vi "DB - [AMS].[Config].[MessageTemplate].vi"(0 "connection reference":T5, 1 "DB Connection":T6={"Open"=TRUE, "Close"=TRUE}, 2 "Simulate Parameters":T1={"Simulate Send SMS"=TRUE, "Simulate Stringx [Unicode]"=FALSE, "Simulate Send Email"=FALSE, "Simulate Email Fail"=FALSE, "Simulate SMS Fail"=FALSE}, 3 "AMS General Settings":T2, 5 "AMS.Execute.Message":string[](array[string]), 9 "AMS Execute Message ColNames":T4[](array[typedef])=[enum."[MessageNo]", enum."[LanguageId]", enum."[SoftwareSolutionId]", enum."[SoftwareSolutionName]", enum."[PlantId]", enum."[SystemId]", enum."[StationId]", enum."[MessageLogNo]", enum."[ReceivedOn]", enum."[MessageCode]", enum."[ShortDescription]", enum."[Message]", enum."[SmsMessage]", enum."[TransactionNo]", enum."[TransactionRunNo]", enum."[MessageInitiator]", enum."[Remarks]", enum."[MsgCreatedOn]", enum."[IsToSendSms]", enum."[IsToSendEmail]", enum."[SmsContent]", enum."[EmailContent]", enum."[MobileNos]", enum."[EmailAddresses]", enum."[LastAttemptedCommMed]", enum."[LastAttemptedNo]", enum."[IsSmsSent]", enum."[IsEmailSent]", enum."[OverallSentStatus]", enum."[IsArchived]"], 11 "error in (no error)":errorcluster, 12 "[CommMediumId]":string="2", 14 "AMS Configure Parameters":T3) -> (4 "connection reference":T5, 6 "AMS.Config.MessageTemplate":string[](array[string]), 8 "All SMS/Email Delivered OK":bool, 15 "SUMMARY":errorcluster)   [LabVIEW 2013]
uses:
  <vilib>/addons/database/Connection.llb/Conn ObjectReference.ctl
  Controls/DB - OpenClose.ctl
  Controls/DB - [AMS].[Execute].[Message] ColNames.ctl
  Controls/Configure Parameters - AMS.ctl
  Controls/General Settings - AMS.ctl
  Controls/Simulate Parameters - AMS.ctl
  Controls/DB - [AMS].[Execute].[Message] Enum.ctl
  Controls/Global AMS.vi
  Controls/Global SRTRS.vi
  <vilib>/addons/database/Connection.llb/DB Tools Open Connec (String).vi
  tool_Unicode_Convert Unicode to ASCII (Scalar).vi
  <vilib>/addons/database/NI_Database_API.lvlib
panel:
  out "Email Subject (ASCII)":string
  out "AMS.Execute.MessageProcessLog 2":errorcluster
  out "AMS.Execute.Message":errorcluster
  out "AMS.Execute.SmsRefNoLogRelation":errorcluster
  out "[MessageNo]":string
  out "Final Message Delivered OK":bool[](array[boolean])
  in  "AMS.Execute.SmsRefNoLogRelation":string="AMS.Execute.SmsRefNoLogRelation"
  out "AMS.Execute.MessageProcessLog":errorcluster
  in  "AMS.Execute.MessageProcessLog":string="AMS.Execute.MessageProcessLog"
  out "SMS":errorcluster
  out "Email":errorcluster
  out "Message Delivered OK":bool
  in  "Simulate Stringx [Unicode]":string="°e RaW"
  out "SMSString":string
  out "[MessageTemplate.Subject] Unicode":string
  out "EmailAddresses":string[](array[string])
  out "AMS.Config.CommDevice":errorcluster
  out "AMS.Config.CommDeviceCountry":errorcluster
  in  "AMS.Config.CommDevice":string="AMS.Config.CommDevice"
  out "MobileNo/Email, CommDeviceId":string[][](array[string])
  out "MobileNos":string[](array[string])
  out "AMS.Config.CommDeviceCountry":string[][](array[string])
  in  "AMS.Config.CommDeviceCountry":string="AMS.Config.CommDeviceCountry"
  out "SQL":string[](array[string])
  out "AMS.Config.MessageTemplate":errorcluster
  out "AMS.Config.Language":errorcluster
  out "Stringx [Unicode]":string
  out "[IsUnicode]":bool
  in  "AMS.Config.Language":string="AMS.Config.Language"
  out "[SoftwareSolutionId]":string
  out "Close":errorcluster
  out "[LanguageId]":string
  in  "AMS.Config.MessageTemplate":string="AMS.Config.MessageTemplate"
  out "Connection Information":T7={"Connection "="SQL Server 32bit HPEnvy", "Username"="admin", "Password"="admin123"}
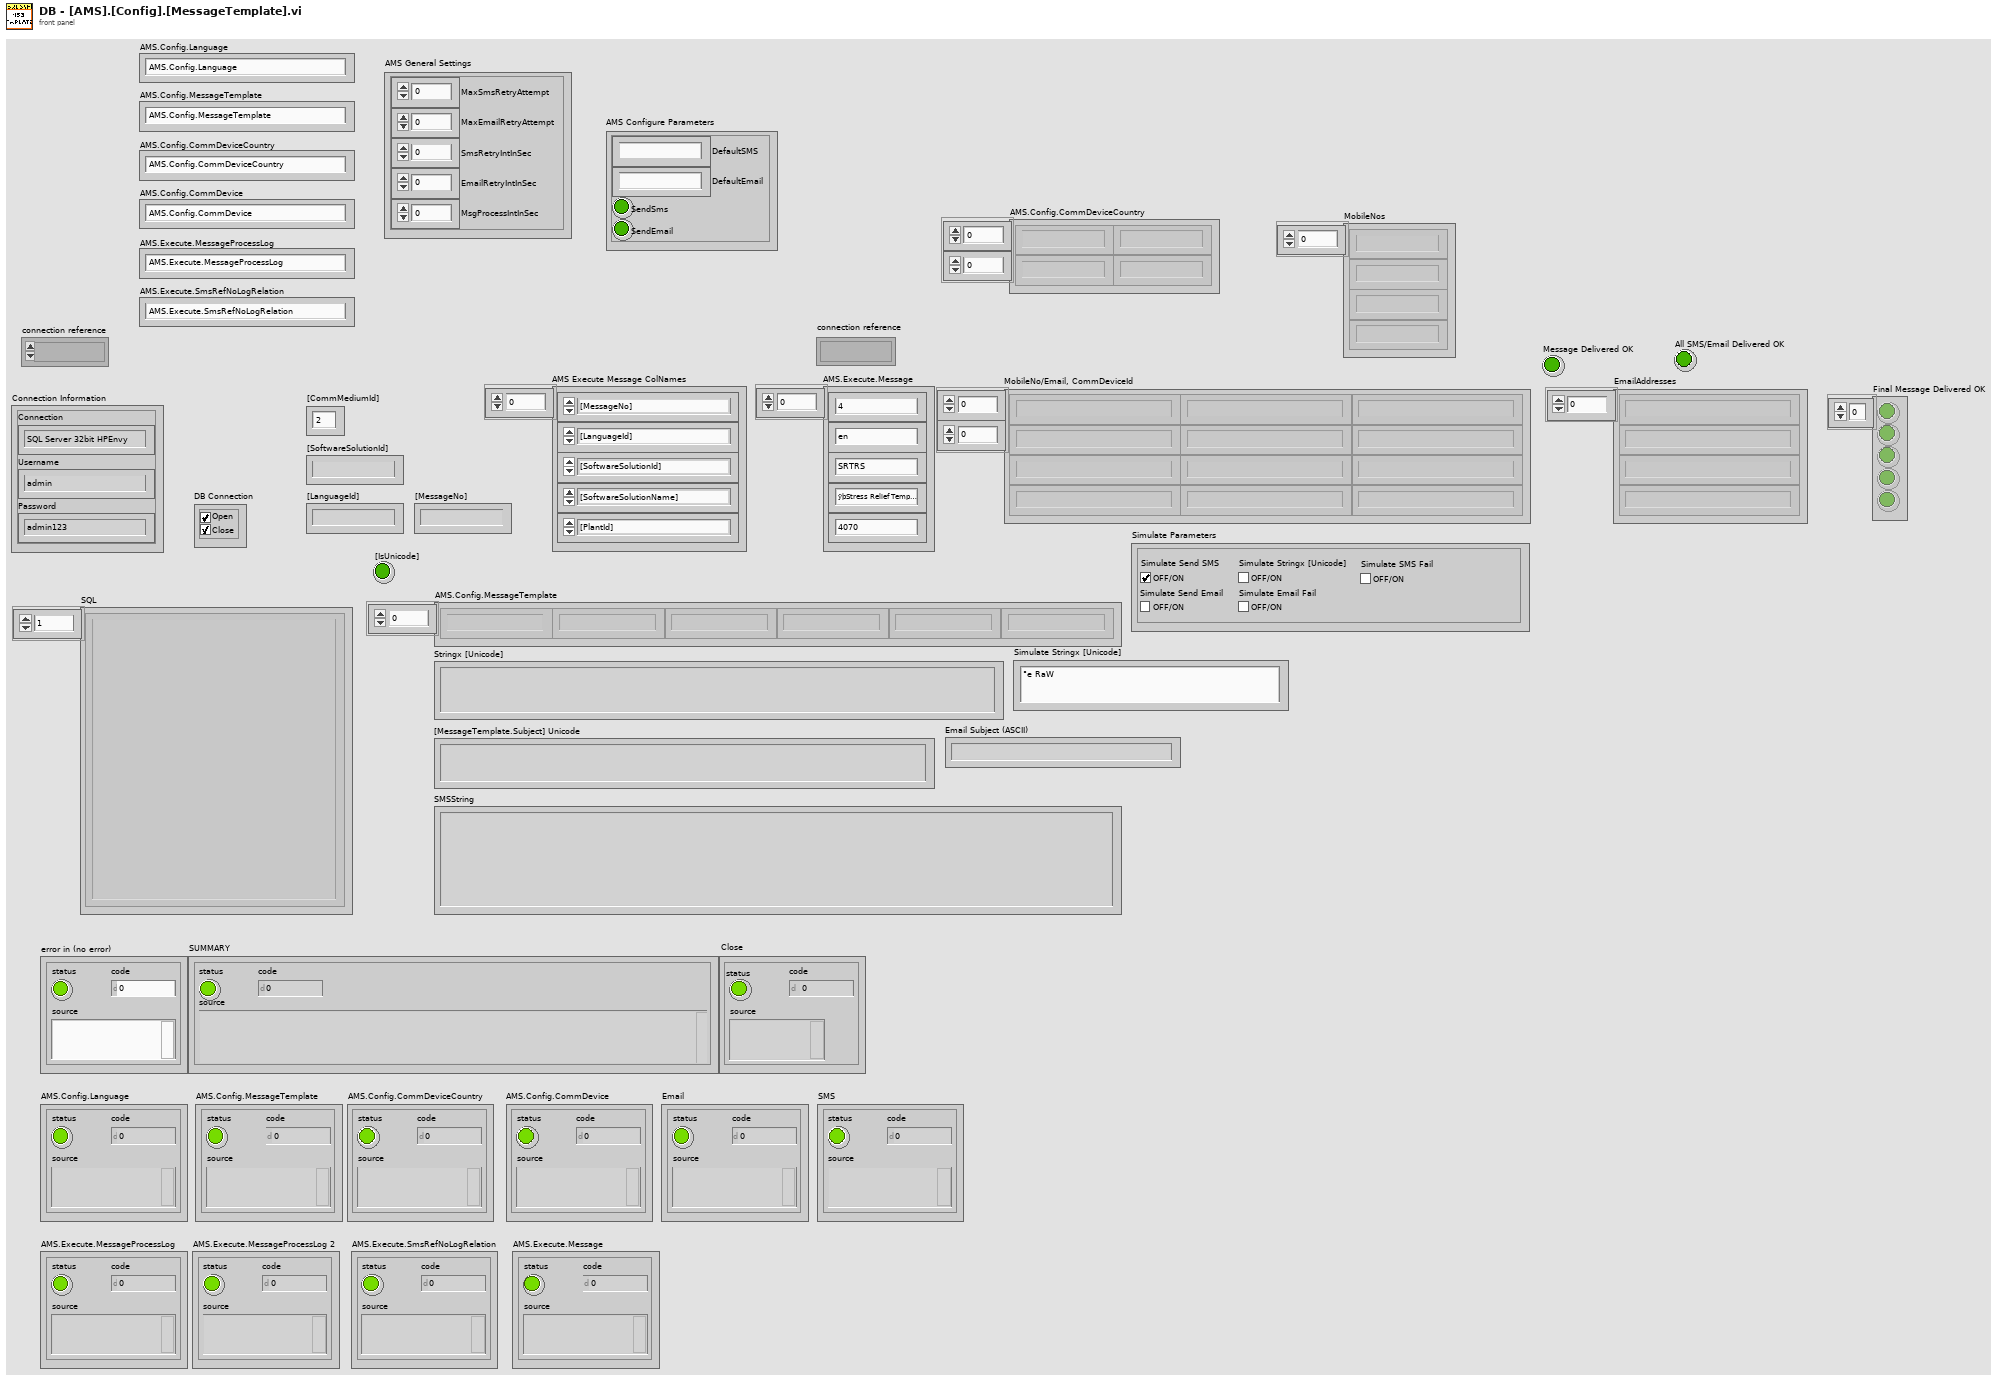
[diagram p1: front panel]
types:
  T1 = typedef "Simulate Parameters - AMS.ctl" = cluster{"Simulate Send SMS":bool, "Simulate Stringx [Unicode]":bool, "Simulate Send Email":bool, "Simulate Email Fail":bool, "Simulate SMS Fail":bool}
  T2 = typedef "General Settings - AMS.ctl" = cluster{"MaxSmsRetryAttempt":i32, "MaxEmailRetryAttempt":i32, "SmsRetryIntInSec":i32, "EmailRetryIntInSec":i32, "MsgProcessIntInSec":i32}
  T3 = typedef "Configure Parameters - AMS.ctl" = cluster{"DefaultSMS":string, "DefaultEmail":string, "SendSms":bool, "SendEmail":bool}
  T4 = typedef "DB - [AMS].[Execute].[Message] ColNames.ctl" = enum16{"[MessageNo]", "[LanguageId]", "[SoftwareSolutionId]", "[SoftwareSolutionName]", "[PlantId]", "[SystemId]", "[StationId]", "[MessageLogNo]", "[ReceivedOn]", "[MessageCode]", "[ShortDescription]", "[Message]", "[SmsMessage]", "[SuppMessage1]", "[SuppMessage2]", "[SuppMessage3]", "[TransactionNo]", "[TransactionRunNo]", "[MessageInitiator]", "[Remarks]", "[MsgCreatedOn]", "[IsToSendSms]", "[IsToSendEmail]", "[IsToSendCommMedium1]", "[IsToSendCommMedium2]", "[SmsContent]", "[EmailContent]", "[CommMed1Content]", "[CommMed2Content]", "[MobileNos]", "[EmailAddresses]", "[CommMedium1Ids]", "[CommMedium2Ids]", "[LastAttemptedCommMed]", "[LastAttemptedNo]", "[LastAttemptedOn]", "[IsSmsSent]", "[IsEmailSent]", "[IsCommMedium1Sent]", "[IsCommMedium2Sent]", "[OverallSentStatus]", "[StatusUpdatedOn]", "[IsArchived]"}
  T5 = typedef "NI_Database_API.lvlib/Conn ObjectReference.ctl" = refnum<k1>
  T6 = typedef "DB - OpenClose.ctl" = cluster{"Open":bool, "Close":bool}
  T7 = cluster{"Connection ":string, "Username":string, "Password":string}
  T8 = typedef "Enum - InteractiveMode-SubVIMode.ctl" = enum16{"Interactive", "subVI Mode"}
  T9 = typedef "Connection Information Cluster.ctl" = cluster{"Connection ":string, "Username":string, "Password":string}
  T10 = typedef "DB - DB.Schema.Table.ctl" = cluster{"DB":string, "Schema":string, "Table":string}
  T11 = typedef "DB - [AMS].[Execute].[Message] Enum.ctl" = enum16{"SELECT", "SELECT (Multi-Conditions)", "UPDATE", "RE-INSERT"}
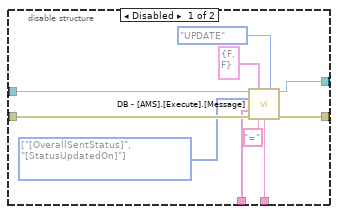
[diagram p2: hidden frame]
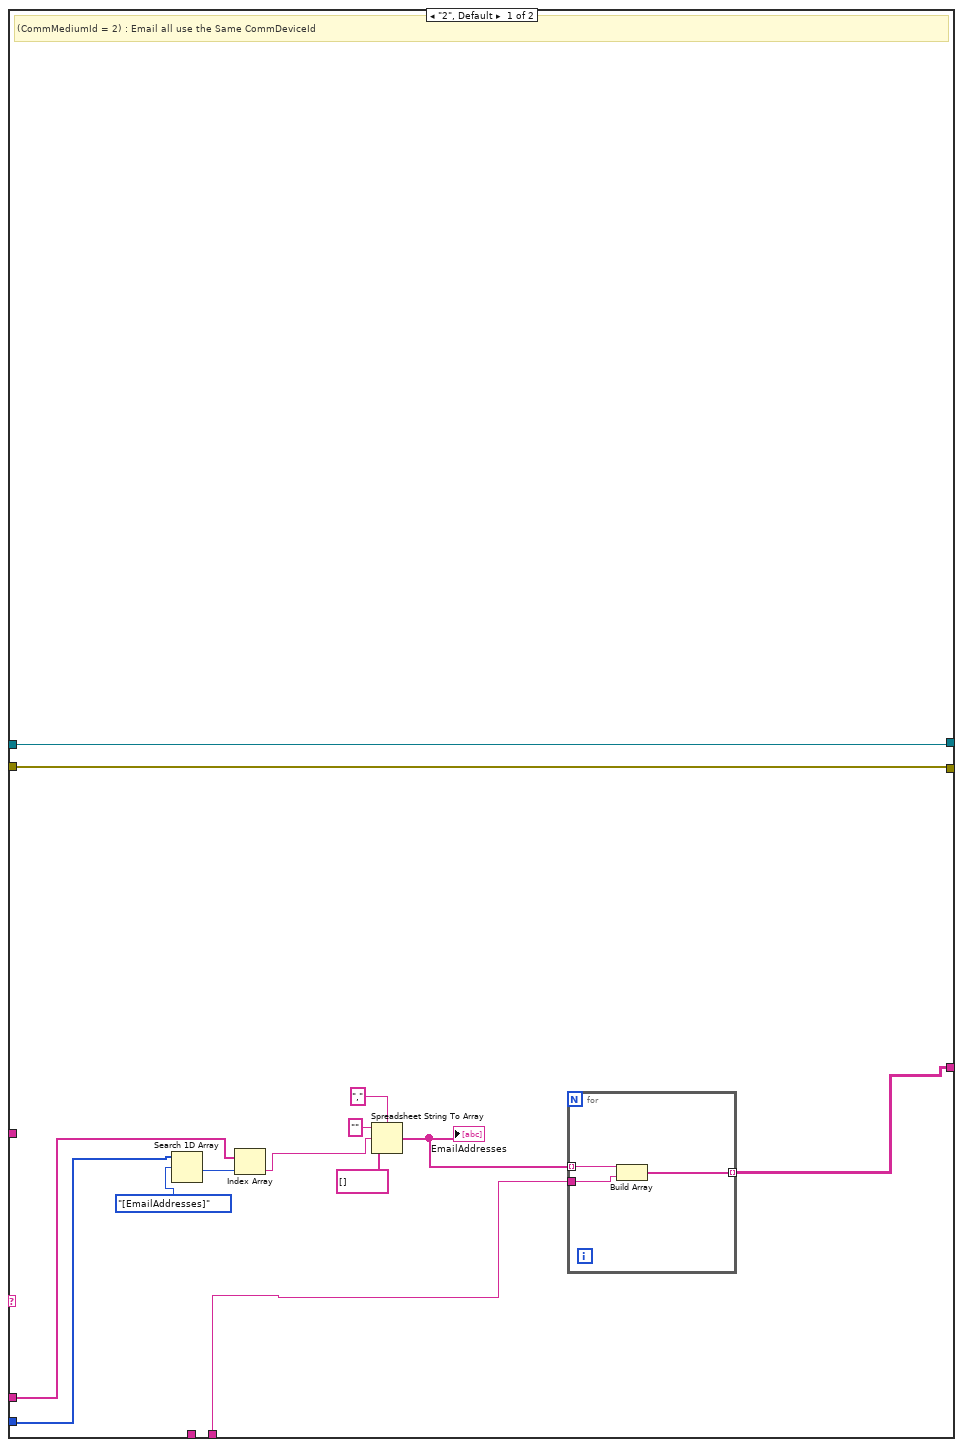
[diagram p3: hidden frame]
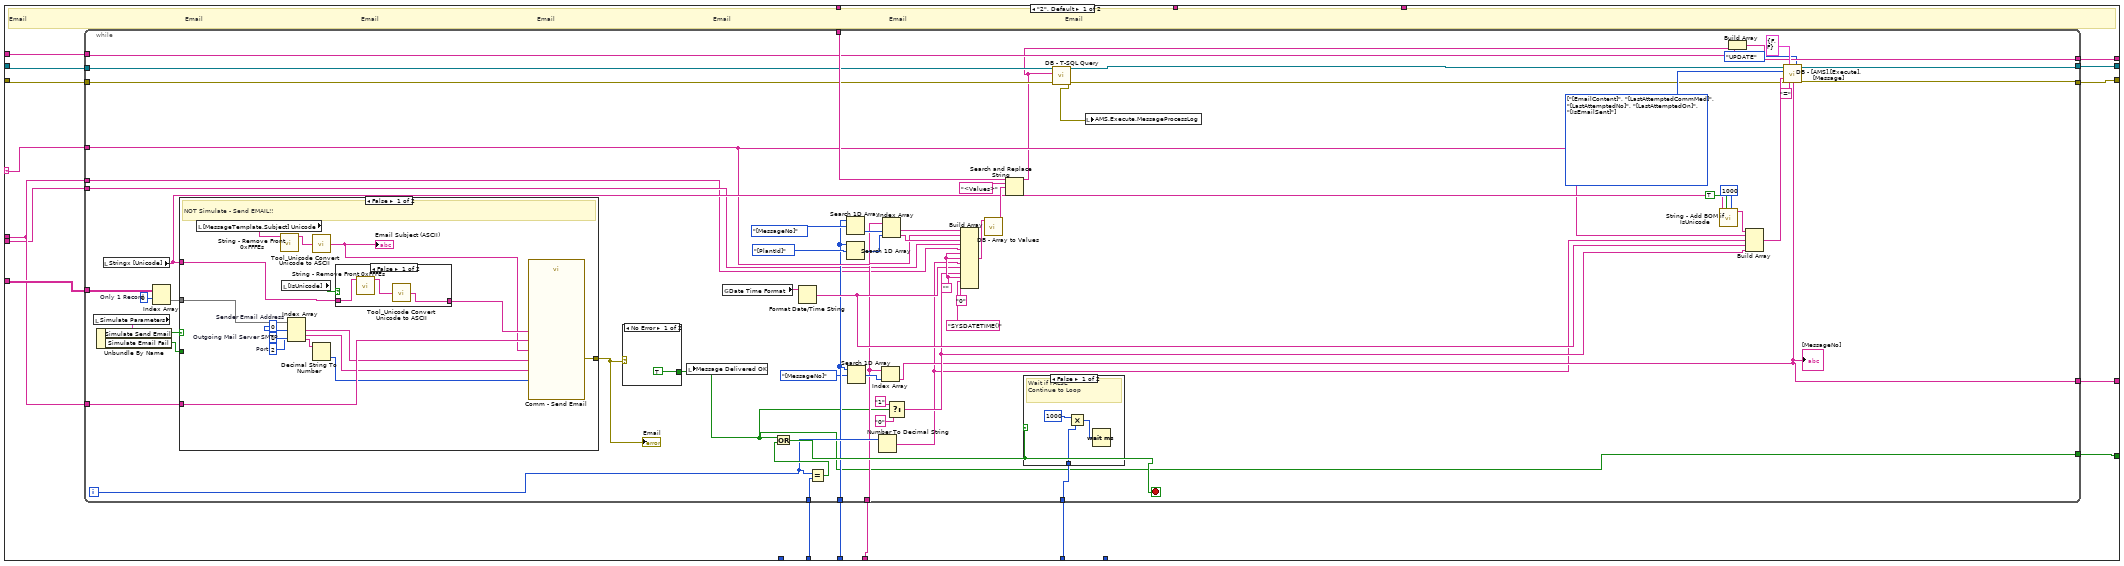
[diagram p4: hidden frame]
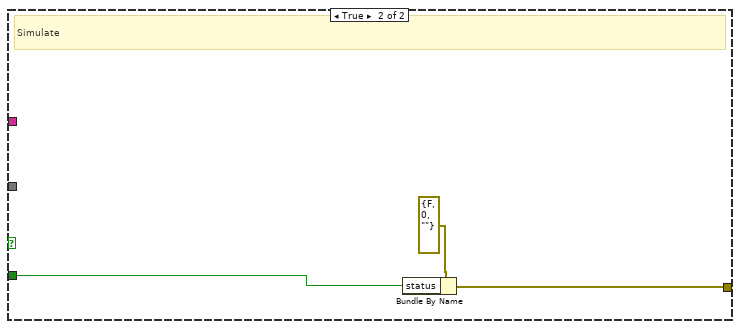
[diagram p6: hidden frame]
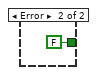
[diagram p8: hidden frame]
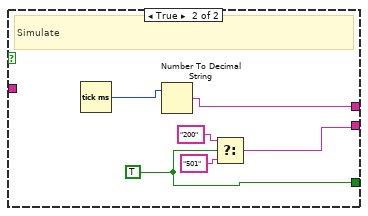
[diagram p10: hidden frame]
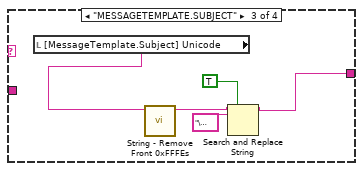
[diagram p13: hidden frame]
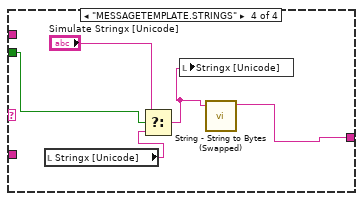
[diagram p14: hidden frame]
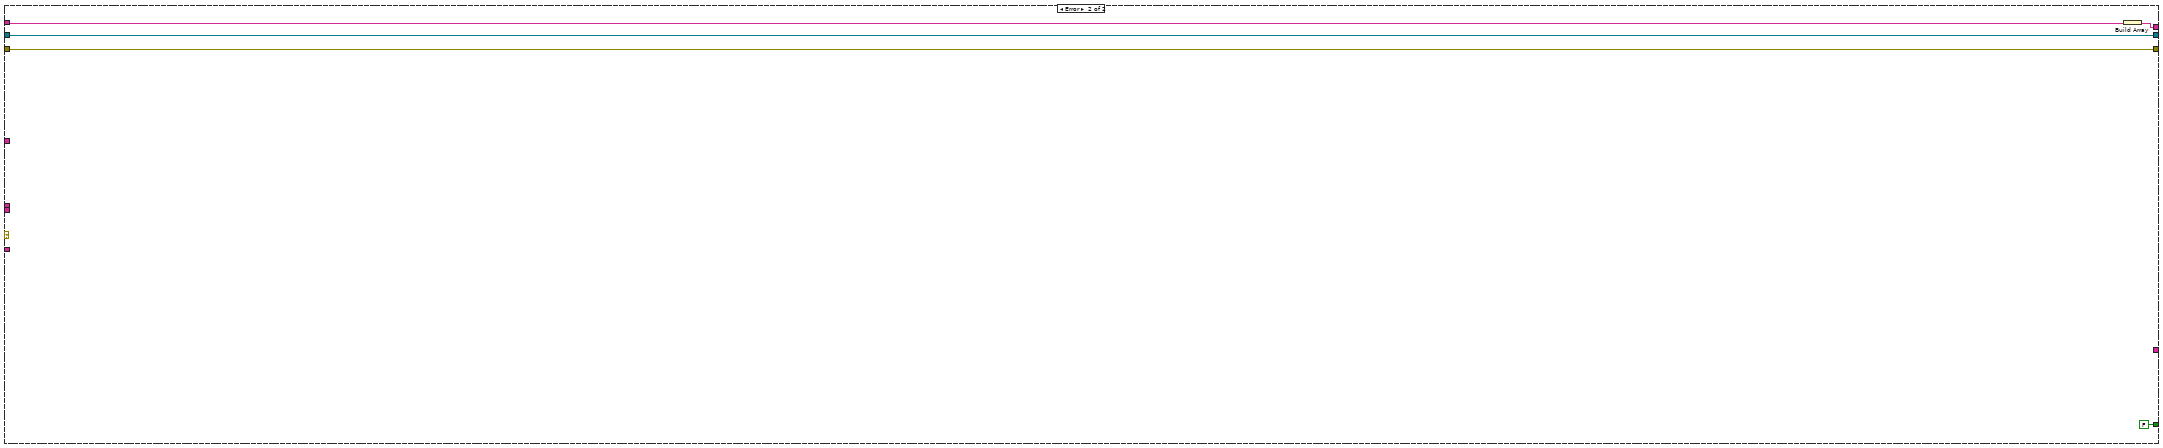
[diagram p15: hidden frame]
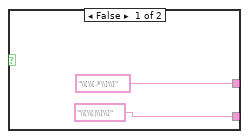
[diagram p16: hidden frame]
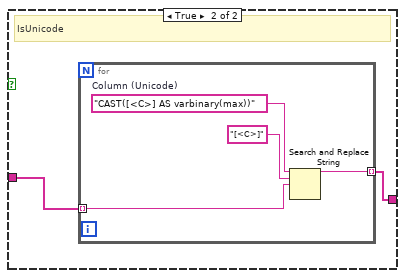
[diagram p18: hidden frame]
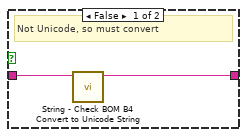
[diagram p20: hidden frame]
diagram:
  w64 = string[] ["[Subject]", "[String1]", "[String2]", "[String3]", "[String4]", "[String5]", "[String6]", "[String7]", "[String8]", "[String9]", "[String10]", "[String11]", "[String12]", "[String13]", "[String14]", "[String15]", "[String16]", "[String17]", "[String18]", "[String19]", "[String20]", "[String21]", "[String22]", "[String23]", "[String24]"]  # AMS.Config.MessageTemplate Columns
  w69 = 0 ("index (row)")
  (unwired) "CAST([<C>] AS varbinary(max))"  # Column (Unicode)
  n1 = call "VI - Interactive or SubVI.vi"() -> ("Mode"=w90:T8)  [unwired: 5 in]
  n2 = case shown="\"subVI Mode\"" w90 {
    tunnel: [w93 "error in (no error)"] -> w89
    frame "Interactive", Default {
      w93 = errorcluster {"status"=FALSE, "code"=0, "source"=""} ("error in (no error)")
      n3 = local write "error in (no error)"(w93) -> ()
    }
    frame "subVI Mode" {
    }
  }
  n4 = global read "Global AMS.vi" "AMS Connection Information"() -> (w82:T9)
  n5 = Unbundle By Name("DB Connection") -> ("Open"=w91:bool, "Close"=w88:bool)
  n6 = case shown="True" w91 {
    tunnel: ["connection reference" w100] -> w77
    tunnel: w89 -> [w95 w99]
    tunnel: [w95 w98] -> w76
    tunnel: w82 -> [_ w97]
    frame False {
      # "Ref Connected"
    }
    frame True {
      # "OPEN"
      n7 = Unbundle By Name(w97) -> ("Connection"=w102:string, "Username"=w103:string, "Password"=w101:string)
      n8 = call-poly <vilib>:"DB Tools Open Connection.vi"("password"=w101, "userID"=w103, "error in (no error)"=w99, "connection information"=w102) -> ("error out"=w98:errorcluster, "connection reference"=w100:T5)  [unwired: 4 in]
      "Connection Information" <- w97
    }
  }
  n9 = Search 1D Array(1D array="AMS Execute Message ColNames", element=DB_-_[AMS].[Execute].[Message]_ColNames."[LanguageId]" ("[AMS].[Execute].[Message] ColNames")) -> (index of element=w48:i32)  [unwired: 1 in]
  n10 = Search 1D Array(1D array="AMS Execute Message ColNames", element=DB_-_[AMS].[Execute].[Message]_ColNames."[SoftwareSolutionId]" ("[AMS].[Execute].[Message] ColNames")) -> (index of element=w46:i32)  [unwired: 1 in]
  n11 = call "DB - Split DB.Schema.Table.vi"("DB.Schema.Table"="AMS.Config.Language") -> ("DB.Schema.Table"=w71:T10)  [unwired: 10 in]
  n12 = Index Array(array="AMS.Execute.Message", index=w48) -> (element=w45:string)
  "[LanguageId]" <- w45
  n13 = Index Array(array="AMS.Execute.Message", index=w46) -> (element=w44:string)
  "[SoftwareSolutionId]" <- w44
  n14 = call "DB - Replace DB.Schema.Table.vi"("DB.Schema.Table"=w71, "string in"="USE [<DB>]\nSELECT [IsUnicode] FROM \n[<Schema>].[<Table>]\nWHERE [LanguageId] = '<L>' " ("T-SQL")) -> ("string out"=w75:string)  [unwired: 8 in, 1 out]
  n15 = Search and Replace String(input string=w75, search string="<L>", replace string=w45) -> (result string=w55:string)  [unwired: 5 in, 3 out]
  n16 = call "DB - T-SQL Query.vi"("error in (no error)"=w76, "T-SQL"=w55, "connection reference"=w77) -> ("error out"=w66:errorcluster, "2D data"=w70:string[][], "connection reference"=w67:T5)  [unwired: 6 in]
  "AMS.Config.Language" <- w66
  n17 = Index Array(array=w70, index (row)=w69, index (col)=w69) -> (element=w68:string)
  n18 = call "DB - Convert BIT Type.vi"("BIT Type (eg Inactive)"=w68) -> ("Boolean"=w3:bool)  [unwired: 2 in, 2 out]
  "[IsUnicode]" <- w3
  n19 = call "DB - Split DB.Schema.Table.vi"("DB.Schema.Table"="AMS.Config.MessageTemplate") -> ("DB.Schema.Table"=w87:T10)  [unwired: 10 in]
  n20 = disable-structure shown="Disabled" {
    disable-tunnel: w3 -> [w104 _]
    frame Disabled {
      (unwired) "\\" ("substring (\"\")")
      n21 = case shown="True" w104 {
        tunnel: ["\\[\\[.*\\]\\]" ("regular expression") "\\[\\\u0000\\[\\\u0000.*\\]\\\u0000\\]\\\u0000" ("regular expression")] -> _
        tunnel: ["\\[\\[|\\]\\]" ("substring (\"\")") "\\[\\\u0000\\[\\\u0000|\\]\\\u0000\\]\\\u0000" ("substring (\"\")")] -> _
        frame False {
        }
        frame True {
          # "Add \\00 behind [ & ] to cater of \\00\nin Unicode"
        }
      }
    }
    frame Enabled {
    }
  }
  n22 = case shown="False" w3 {
    tunnel: w64 -> [w109 w111]
    tunnel: [w109 w110] -> w60
    frame False {
    }
    frame True {
      # "IsUnicode"
      n23 = for {
        tunnel: w111 -> [w113] mode=indexing
        tunnel: [w112] -> w110 mode=indexing
        w115 = "CAST([<C>] AS varbinary(max))"  # Column (Unicode)
        n24 = Search and Replace String(input string=w115, search string="[<C>]", replace string=w113) -> (result string=w112:string)  [unwired: 5 in, 3 out]
      }
    }
  }
  n25 = call "DB - Replace DB.Schema.Table.vi"("DB.Schema.Table"=w87, "string in"="USE [<DB>]\nSELECT TOP 1 <COLUMNS> \nFROM [<Schema>].[<Table>]\nWHERE [CommMediumId] = '<CM>' AND [LanguageId] = '<L>' AND [SoftwareSolutionId] = '<SS>' AND [Inactive] = '0'\n") -> ("string out"=w61:string)  [unwired: 8 in, 1 out]
  n26 = Array To Spreadsheet String(delimiter (Tab)=",", array=w60, 3:"" ("format string")) -> (spreadsheet string=w57:string)
  n27 = Search and Replace String(input string=w61, search string="<COLUMNS>", replace string=w57) -> (result string=w62:string)  [unwired: 5 in, 3 out]
  n28 = Search and Replace String(input string=w62, search string="<CM>", replace string="[CommMediumId]") -> (result string=w84:string)  [unwired: 5 in, 3 out]
  n29 = Search and Replace String(input string=w84, search string="<L>", replace string=w45) -> (result string=w79:string)  [unwired: 5 in, 3 out]
  n30 = Search and Replace String(input string=w79, search string="<SS>", replace string=w44) -> (result string=w54:string)  [unwired: 5 in, 3 out]
  n31 = for {
    tunnel: "AMS Execute Message ColNames" -> [w117] mode=indexing
    tunnel: [w116] -> w50 mode=indexing
    n32 = Format Into String(w117) -> (resulting string=w116:string)  [unwired: 3 in, 1 out]
  }
  n33 = call "DB - T-SQL Query.vi"("error in (no error)"=w66, "T-SQL"=w54, "connection reference"=w67) -> ("error out"=w51:errorcluster, "2D data"=w65:string[][], "connection reference"=w52:T5)  [unwired: 6 in]
  "AMS.Config.MessageTemplate" <- w51
  n34 = Index Array(array=w65, index (row)=0) -> (element=w2:string[])  [unwired: 1 in]
  "AMS.Config.MessageTemplate" <- w2
  n35 = for {
    tunnel: w2 -> [w123] mode=indexing
    tunnel: w50 -> [w129]
    tunnel: "AMS.Execute.Message" -> [w127]
    tunnel: w3 -> [w126]
    shift-right: [w125] -> w56
    shift-left: "" -> [w122]
    i -> [w124]
    n36 = call "String - Search for [[  ]].vi"("String"=w123, "Strip \\00 (Unicode)"=w126) -> ("after substring"=w118:string, "before substring"=w119:string, "matched string"=w128:string, "Found"=w130:bool)  [unwired: 6 in]
    n37 = case shown="False" w130 {
      tunnel: w129 -> [_ w150]
      tunnel: w128 -> [_ w147]
      tunnel: w127 -> [_ w148]
      tunnel: w123 -> [w133 _]
      tunnel: [w132 w143] -> w121
      tunnel: w126 -> [w134 _]
      tunnel: w119 -> [_ w142]
      tunnel: w118 -> [_ w141]
      tunnel: [w132 w138] -> _
      frame False {
        # "Not [[ColName]], direct CONCAT"
        n38 = case shown="True" w134 {
          tunnel: w133 -> [w136 w137]
          tunnel: [w135 w137] -> w132
          frame False {
            # "Not Unicode, so must convert"
            n39 = call "String - Check BOM B4 Convert to Unicode String.vi"("Check 0xFFEE"=w136) -> ("Convert ASCII to Unicode"=w135:string)  [unwired: 10 in]
          }
          frame True {
            # "IsUnicode already"
          }
        }
      }
      frame True {
        # "[[ColName]] Found\nGet Column Index\nGet Value"
        n40 = Concatenate Strings "Join Back [ ] to search"("[" ("string"), w147, "]" ("string")) -> (w144:string)
        n41 = Search 1D Array(1D array=w150, element=w144) -> (index of element=w149:i32)  [unwired: 1 in]
        n42 = Index Array(array=w148, index=w149) -> (element=w140:string)
        n43 = Concatenate Strings "Join Back pre [ ] post"(w142, w140, w141) -> (w139:string)
        n44 = call "String - Check BOM B4 Convert to Unicode String.vi"("Check 0xFFEE"=w139) -> ("Convert ASCII to Unicode"=w138:string)  [unwired: 10 in]
        n45 = call "String - Check BOM B4 Convert to Unicode String.vi"("Check 0xFFEE"=w140) -> ("Convert ASCII to Unicode"=w143:string)  [unwired: 10 in]
      }
    }
    n46 = call "String - Remove Front 0xFFFEs.vi"("Sting IN"=w121) -> ("String OUT"=w120:string)  [unwired: 10 in]
    n47 = Concatenate Strings(w122, w120) -> (w125:string)
    n48 = case shown="0" w124 {
      tunnel: w120 -> [w131 _]
      frame 0 {
        "[MessageTemplate.Subject] Unicode" <- w131
      }
      frame 1, Default {
      }
    }
  }
  "Stringx [Unicode]" <- w56
  n49 = control-ref of="AMS.Config.MessageTemplate"() -> (w4:refnum<vi>)
  n50 = call "Tool_Unicode Update String Array (1D).vi"("Interpret as Unicode (T)"=w3, "Value"=w2, "String Array (1D) Ref"=w4) -> ()  [unwired: 5 in, 2 out]
  n51 = Search 1D Array(1D array="AMS Execute Message ColNames", element=DB_-_[AMS].[Execute].[Message]_ColNames."[PlantId]" ("[AMS].[Execute].[Message] ColNames")) -> (index of element=w31:i32)  [unwired: 1 in]
  n52 = Index Array(array="AMS.Execute.Message", index=w31) -> (element=w30:string)
  n53 = Unbundle By Name("AMS Configure Parameters") -> ("DefaultSMS"=w27:string, "DefaultEmail"=w26:string)
  n54 = case "[CommMediumId]" shown="\"1\"" "[CommMediumId]" {
    tunnel: w52 -> [w162 w190]
    tunnel: w51 -> [w163 w189]
    tunnel: "AMS.Execute.Message" -> [w160 w176]
    tunnel: [w152 w175] -> w43
    tunnel: [w162 w174] -> w34
    tunnel: [w163 w173] -> w33
    tunnel: w30 -> [_ w170]
    tunnel: "AMS Execute Message ColNames" -> [w159 w168]
    tunnel: w27 -> [_ w167]
    tunnel: w26 -> [w151 _]
    frame "2", Default {
      # "(CommMediumId = 2) : Email all use the Same CommDeviceId"
      n55 = Search 1D Array(1D array=w159, element=DB_-_[AMS].[Execute].[Message]_ColNames."[EmailAddresses]" ("[AMS].[Execute].[Message] ColNames")) -> (index of element=w161:i32)  [unwired: 1 in]
      n56 = Index Array(array=w160, index=w161) -> (element=w154:string)
      n57 = Spreadsheet String To Array(delimiter (Tab)=",", format string="", spreadsheet string=w154, array type (2D Dbl)=string[] []) -> (array=w153:string[])
      "EmailAddresses" <- w153
      n58 = for {
        tunnel: w153 -> [w166] mode=indexing
        tunnel: w151 -> [w165]
        tunnel: [w164] -> w152 mode=indexing
        n59 = Build Array(w166, w165) -> (w164:string[])
      }
    }
    frame "1" {
      w178 = 1  # [CommDeviceId]
      w187 = 0  # [CountryCode]
      # "(CommMediumId = 1) SMS, Choose a diferent CommDeviceId according to CountryCode Match"
      n60 = Search 1D Array(1D array=w168, element=DB_-_[AMS].[Execute].[Message]_ColNames."[MobileNos]" ("[AMS].[Execute].[Message] ColNames")) -> (index of element=w171:i32)  [unwired: 1 in]
      n61 = call "DB - Split DB.Schema.Table.vi"("DB.Schema.Table"="AMS.Config.CommDeviceCountry") -> ("DB.Schema.Table"=w191:T10)  [unwired: 10 in]
      n62 = Index Array(array=w176, index=w171) -> (element=w169:string)
      n63 = call "DB - Replace DB.Schema.Table.vi"("DB.Schema.Table"=w191, "string in"="USE [<DB>]\nSELECT \n      [CountryCode], [CommDeviceId]\n      \n  FROM [<Schema>].[<Table>] WHERE [Inactive] = '0' AND [PlantId] = '<P>'") -> ("string out"=w180:string)  [unwired: 8 in, 1 out]
      n64 = Spreadsheet String To Array(delimiter (Tab)=",", format string="", spreadsheet string=w169, array type (2D Dbl)=string[] []) -> (array=w183:string[])
      "MobileNos" <- w183
      n65 = Search and Replace String(input string=w180, search string="<P>", replace string=w170) -> (result string=w179:string)  [unwired: 5 in, 3 out]
      n66 = call "DB - T-SQL Query.vi"("error in (no error)"=w189, "T-SQL"=w179, "connection reference"=w190) -> ("error out"=w173:errorcluster, "2D data"=w188:string[][], "connection reference"=w174:T5)  [unwired: 6 in]
      "AMS.Config.CommDeviceCountry" <- w188
      "AMS.Config.CommDeviceCountry" <- w173
      n67 = Index Array(array=w188, index (col) #1=w187, index (col) #2=w178) -> (element #1=w186:string[], element #2=w177:string[])  [unwired: 2 in]
      n68 = for {
        tunnel: w186 -> [w198]
        tunnel: w183 -> [w197] mode=indexing
        tunnel: w177 -> [w196]
        tunnel: w167 -> [w195]
        tunnel: [w194] -> w175 mode=indexing
        # "Each MobileNos OR EmailAddress"
        n69 = for {
          tunnel: w198 -> [w205] mode=indexing
          tunnel: w197 -> [w202]
          tunnel: w196 -> [w203] mode=indexing
          tunnel: w195 -> [w200]
          tunnel: [w199] -> w194
          # "If [CountryCode] Found, use [CommDeviceCountry] otherwise\nuse AMS.Config.Parameter.DefaultSMS"
          n70 = String Length(string=w205) -> (length=w207:i32)
          n71 = String Subset(string=w202, length (rest)=w207) -> (substring=w206:string)  [unwired: 1 in]
          n72 = Equal?(x=w206, y=w205) -> (x = y?=w204:bool)
          n73 = Select(t=w203, s=w204, f=w200) -> (s? t:f=w201:string)
          n74 = Build Array(w202, w201) -> (w199:string[])
        }
      }
    }
  }
  "MobileNo/Email, CommDeviceId" <- w43
  n75 = call "DB - Split DB.Schema.Table.vi"("DB.Schema.Table"="AMS.Config.CommDevice") -> ("DB.Schema.Table"=w40:T10)  [unwired: 10 in]
  n76 = call "DB - Replace DB.Schema.Table.vi"("DB.Schema.Table"=w40, "string in"="USE [<DB>]\n\nSELECT \n       [String1]\n      ,[String2]\n      ,[String3]\n      ,[String4]\n      ,[String5]\n      ,[String6]\n      ,[String7]\n      ,[String8]\n      ,[String9]\n      ,[String10]\n      ,[String11]\n      ,[String12]\n      ,[SmsProcessStatusCode]\n      ,[SmsDeliveredStatusCode]\n    FROM [<Schema>].[<Table>]\nWHERE  [PlantId] = '<P>' AND [CommDeviceId] = '<CD>' AND [CommMediumId] = '<CM>' AND [Inactive] = '0'\n") -> ("string out"=w42:string)  [unwired: 8 in, 1 out]
  n77 = Search and Replace String(input string=w42, search string="<P>", replace string=w30) -> (result string=w36:string)  [unwired: 5 in, 3 out]
  n78 = Search and Replace String(input string=w36, search string="<CM>", replace string="[CommMediumId]") -> (result string=w35:string)  [unwired: 5 in, 3 out]
  n79 = call "DB - Split DB.Schema.Table.vi"("DB.Schema.Table"="AMS.Execute.MessageProcessLog") -> ("DB.Schema.Table"=w24:T10)  [unwired: 10 in]
  n80 = call "DB - Replace DB.Schema.Table.vi"("DB.Schema.Table"=w24, "string in"="USE [<DB>]\n\nINSERT INTO [<Schema>].[<Table>]\n           ([MessageNo]\n           ,[CommMediumId]\n           ,[PlantId]\n           ,[CommDeviceId]\n           ,[SentTo]\n           ,[MessageRefNo]\n           ,[StatusId]\n           ,[RetryNo]\n           ,[ProcessedOn]\n           ,[IsSentSuccess]\n           ,[AcknowledgedOn]\n           ,[CreatedOn]\n           ,[IsArchived])\n     VALUES\n (<Values>)\n") -> ("string out"=w23:string)  [unwired: 8 in, 1 out]
  n81 = call "DB - Split DB.Schema.Table.vi"("DB.Schema.Table"="AMS.Execute.MessageProcessLog") -> ("DB.Schema.Table"=w20:T10)  [unwired: 10 in]
  n82 = call "DB - Replace DB.Schema.Table.vi"("DB.Schema.Table"=w20, "string in"="USE [<DB>]\n\nSELECT TOP 1 [LogNumber] \nFROM [<Schema>].[<Table>]\nWHERE [MessageRefNo] = '<MRN>' AND [IsArchived] = '0'\n") -> ("string out"=w18:string)  [unwired: 8 in, 1 out]
  n83 = call "DB - Split DB.Schema.Table.vi"("DB.Schema.Table"="AMS.Execute.SmsRefNoLogRelation") -> ("DB.Schema.Table"=w17:T10)  [unwired: 10 in]
  n84 = call "DB - Replace DB.Schema.Table.vi"("DB.Schema.Table"=w17, "string in"="USE [AMS]\n\nINSERT INTO [Execute].[SmsRefNoLogRelation]\n           ([PlantId]\n           ,[CommDeviceId]\n           ,[MessageRefNo]\n           ,[LogNumber]\n           ,[InActive])\n     VALUES\n          (<Values>)\n") -> ("string out"=w15:string)  [unwired: 8 in, 1 out]
  n85 = for {
    tunnel: w43 -> [w227] mode=indexing
    shift-right: [w215] -> w11
    shift-left: w33 -> [w231]
    tunnel: w35 -> [w229]
    tunnel: w34 -> [w228]
    tunnel: [w216] -> w13
    tunnel: [w209] -> w7 mode=concatenating
    tunnel: "[CommMediumId]" -> [w224]
    tunnel: w23 -> [w221]
    tunnel: "AMS.Execute.Message" -> [w217]
    tunnel: "AMS Execute Message ColNames" -> [w218]
    tunnel: w18 -> [w213]
    tunnel: w15 -> [w212]
    tunnel: [w211] -> w9 mode=indexing
    tunnel: [w208] -> w5
    w225 = 1  # CommDeviceId
    w226 = 0  # MobileNo/Email
    # "Each MobileNos"
    n86 = Index Array(array=w227, index #1=w226, index #2=w225) -> (element #1=w222:string, element #2=w214:string)
    n87 = Search and Replace String(input string=w229, search string="<CD>", replace string=w214) -> (result string=w210:string)  [unwired: 5 in, 3 out]
    n88 = call "DB - T-SQL Query.vi"("error in (no error)"=w231, "T-SQL"=w210, "connection reference"=w228) -> ("error out"=w219:errorcluster, "2D data"=w223:string[][], "connection reference"=w220:T5)  [unwired: 6 in]
    "AMS.Config.CommDevice" <- w219
    n89 = case shown="No Error" w219 {
      tunnel: w224 -> [w253 _]
      tunnel: w223 -> [w252 _]
      tunnel: w222 -> [w251 _]
      tunnel: w221 -> [w245 _]
      tunnel: w220 -> [w244 w513]
      tunnel: w219 -> [w243 w512]
      tunnel: w218 -> [w242 _]
      tunnel: w217 -> [w241 _]
      tunnel: [w240 w513] -> w216
      tunnel: [w239 w512] -> w215
      tunnel: w214 -> [w238 _]
      tunnel: w213 -> [w237 _]
      tunnel: w212 -> [w236 _]
      tunnel: [w235 FALSE] -> w211
      tunnel: w210 -> [w234 w510]
      tunnel: [w233 w509] -> w209
      tunnel: [w232 _] -> w208
      frame No Error {
        n90 = Unbundle By Name("AMS General Settings") -> ("MaxSmsRetryAttempt"=w249:i32, "MaxEmailRetryAttempt"=w246:i32, "SmsRetryIntInSec"=w248:i32, "EmailRetryIntInSec"=w247:i32)
        n91 = case "[CommMediumId]" shown="\"1\"" w253 {
          selector: w253 -> [w266 w372]
          tunnel: w252 -> [w270 w387]
          tunnel: w251 -> [w265 w368]
          tunnel: w249 -> [_ w379]
          tunnel: w248 -> [_ w378]
          tunnel: w247 -> [w269 _]
          tunnel: w246 -> [w268 _]
          tunnel: w245 -> [w267 w377]
          tunnel: w244 -> [w263 w376]
          tunnel: w243 -> [w262 w375]
          tunnel: w242 -> [w259 w374]
          tunnel: w241 -> [w258 w373]
          tunnel: [w261 w371] -> w240
          tunnel: [w260 w370] -> w239
          tunnel: w238 -> [w264 w369]
          tunnel: w237 -> [_ w367]
          tunnel: w236 -> [_ w366]
          tunnel: [w257 w365] -> w235
          tunnel: w234 -> [w256 w364]
          tunnel: [w255 w363] -> w233
          tunnel: [w254 w362] -> w232
          frame "2", Default {
            # "Email                                                                               Email                                                                               Email                                                                               Email                                                                               Email                                                                               Email                                                                               Email"
            n92 = while {
              tunnel: w270 -> [w329]
              tunnel: w265 -> [w326]
              tunnel: w269 -> [w325]
              tunnel: w268 -> [w324]
              tunnel: w267 -> [w308]
              tunnel: w266 -> [w291]
              tunnel: w265 -> [w271]
              tunnel: w264 -> [w272]
              tunnel: w263 -> [w307]
              tunnel: w262 -> [w306]
              tunnel: [w294] -> w261
              tunnel: [w293] -> w260
              tunnel: w259 -> [w288]
              tunnel: w258 -> [w285]
              tunnel: [w282] -> w257
              tunnel: w256 -> [w281]
              tunnel: [w279] -> w255
              tunnel: [w277] -> w254
              i -> [w305]
              stop <- w322 stop-if-true
              w301 = T4[] [enum."[EmailContent]", enum."[LastAttemptedCommMed]", enum."[LastAttemptedNo]", enum."[LastAttemptedOn]", enum."[IsEmailSent]"] items=["[MessageNo]", "[LanguageId]", "[SoftwareSolutionId]", "[SoftwareSolutionName]", "[PlantId]", "[SystemId]", "[StationId]", "[MessageLogNo]", "[ReceivedOn]", "[MessageCode]", "[ShortDescription]", "[Message]", "[SmsMessage]", "[SuppMessage1]", "[SuppMessage2]", "[SuppMessage3]", "[TransactionNo]", "[TransactionRunNo]", "[MessageInitiator]", "[Remarks]", "[MsgCreatedOn]", "[IsToSendSms]", "[IsToSendEmail]", "[IsToSendCommMedium1]", "[IsToSendCommMedium2]", "[SmsContent]", "[EmailContent]", "[CommMed1Content]", "[CommMed2Content]", "[MobileNos]", "[EmailAddresses]", "[CommMedium1Ids]", "[CommMedium2Ids]", "[LastAttemptedCommMed]", "[LastAttemptedNo]", "[LastAttemptedOn]", "[IsSmsSent]", "[IsEmailSent]", "[IsCommMedium1Sent]", "[IsCommMedium2Sent]", "[OverallSentStatus]", "[StatusUpdatedOn]", "[IsArchived]"] ("AMS Execute Message ColNames")
              w303 = ""
              w328 = 0  # Only 1 Record
              n93 = local read "Simulate Parameters"() -> (w276:T1)
              n94 = Unbundle By Name(w276) -> ("Simulate Send Email"=w275:bool, "Simulate Email Fail"=w274:bool)
              n95 = local read "Stringx [Unicode]"() -> (w292:string)
              n96 = Index Array(array=w329, index (row)=w328) -> (element=w327:string[])  [unwired: 1 in]
              n97 = case shown="False" w275 {
                tunnel: w327 -> [w345 _]
                tunnel: w326 -> [w341 _]
                tunnel: [w336 w351] -> w283
                tunnel: w292 -> [w334 _]
                tunnel: w274 -> [_ w350]
                frame False {
                  w342 = 2  # Port
                  w343 = 1  # Outgoing Mail Server SMTP
                  w344 = 0  # Sender Email Address
                  # "NOT Simulate - Send EMAIL!!"
                  n98 = local read "[MessageTemplate.Subject] Unicode"() -> (w331:string)
                  n99 = call "String - Remove Front 0xFFFEs.vi"("Sting IN"=w331) -> ("String OUT"=w332:string)  [unwired: 10 in]
                  n100 = local read "[IsUnicode]"() -> (w335:bool)
                  n101 = Index Array(array=w345, index #1=w344, index #2=w343, index #3=w342) -> (element #1=w338:string, element #2=w337:string, element #3=w340:string)
                  n102 = call-poly "Tool_Unicode Convert Unicode to ASCII.vi"("Unicode"=w332) -> ("ASCII"=w330:string)  [unwired: 4 in]
                  "Email Subject (ASCII)" <- w330
                  n103 = Decimal String To Number(string=w340) -> (number=w339:i32)  [unwired: 2 in, 1 out]
                  n104 = case shown="False" w335 {
                    tunnel: w334 -> [w348 w349]
                    tunnel: [w346 w349] -> w333
                    frame False {
                      n105 = call "String - Remove Front 0xFFFEs.vi"("Sting IN"=w348) -> ("String OUT"=w347:string)  [unwired: 10 in]
                      n106 = call-poly "Tool_Unicode Convert Unicode to ASCII.vi"("Unicode"=w347) -> ("ASCII"=w346:string)  [unwired: 4 in]
                    }
                    frame True {
                    }
                  }
                  n107 = call "Comm - Send Email.vi"("Outgoing Mail Server (SMTP)"=w337, "Sender's Email Address"=w338, "Port"=w339, "Message"=w333, "Subject"=w330, "Recipients"=w341) -> ("error out"=w336:errorcluster)  [unwired: 5 in]
                }
                frame True {
                  # "Simulate"
                  n108 = Bundle By Name(cluster=errorcluster {"status"=FALSE, "code"=0, "source"=""} ("error out"), "status"=w350) -> (w351:errorcluster)
                }
              }
              "Email" <- w283
              n109 = case shown="No Error" w283 {
                tunnel: [TRUE FALSE] -> w282
                frame No Error {
                }
                frame Error {
                }
              }
              n110 = local write "Message Delivered OK"(w282) -> ()
              n111 = global read "Global AMS.vi" "Date Time Format"() -> (w312:string)
              n112 = Format Date/Time String(time format string (%c)=w312) -> (date/time string=w290:string)  [unwired: 2 in]
              n113 = Equal?(x=w305, y=w324) -> (x = y?=w323:bool)
              n114 = Or(x=w282, y=w323) -> (x .or. y?=w322:bool)
              n115 = Search 1D Array(1D array=w288, element=DB_-_[AMS].[Execute].[Message]_ColNames."[MessageNo]" ("[AMS].[Execute].[Message] ColNames")) -> (index of element=w319:i32)  [unwired: 1 in]
              n116 = Search 1D Array(1D array=w288, element=DB_-_[AMS].[Execute].[Message]_ColNames."[PlantId]" ("[AMS].[Execute].[Message] ColNames")) -> (index of element=w314:i32)  [unwired: 1 in]
              n117 = Search 1D Array(1D array=w288, element=DB_-_[AMS].[Execute].[Message]_ColNames."[MessageNo]" ("[AMS].[Execute].[Message] ColNames")) -> (index of element=w286:i32)  [unwired: 1 in]
              n118 = Number To Decimal String(number=w305) -> (decimal integer string=w273:string)  [unwired: 1 in]
              n119 = Index Array(array=w285, index=w286) -> (element=w277:string)
              "[MessageNo]" <- w277
              n120 = Index Array(array=w285, index #1=w319, index #2=w314) -> (element #1=w317:string, element #2=w313:string)
              n121 = Select(t="1", s=w282, f="0") -> (s? t:f=w289:string)
              n122 = Build Array(w317, w291, w313, w272, w271, w303, w303, w273, w290, w289, w303, "SYSDATETIME()", "0") -> (w315:string[])
              n123 = call "DB - Array to Values.vi"("Array (0xFFFE autodetect)"=w315) -> ("<Values>"=w316:string)  [unwired: 10 in]
              n124 = Search and Replace String(input string=w308, search string="<Values>", replace string=w316) -> (result string=w280:string)  [unwired: 5 in, 3 out]
              n125 = case shown="False" w322 {
                tunnel: w325 -> [w354 _]
                frame False {
                  # "Wait if FALSE\nContinue to Loop"
                  n126 = Multiply(x=1000, y=w354) -> (x*y=w355:i32)
                  n127 = Wait (ms)(milliseconds to wait=w355) -> ()  [unwired: 1 out]
                }
                frame True {
                  # "Stop Loop"
                }
              }
              n128 = call "DB - T-SQL Query.vi"("error in (no error)"=w306, "T-SQL"=w280, "connection reference"=w307) -> ("error out"=w295:errorcluster, "connection reference"=w296:T5)  [unwired: 6 in, 1 out]
              n129 = local write "AMS.Execute.MessageProcessLog"(w295) -> ()
              n130 = call "String - Add BOM if IsUnicode.vi"("target length (65535)"=1000, "Input is Unicode (varbinary)?"=TRUE ("IsUnicode?"), "String IN"=w292) -> ("BOM Added"=w300:string)  [unwired: 8 in]
              n131 = Build Array(w281, w280) -> (w279:string[])
              n132 = Build Array(w300, w291, w273, w290, w289) -> (w297:string[])
              n133 = call "DB - [AMS].[Execute].[Message].vi"("connection reference"=w296, "DB Connection"=T6 {"Open"=FALSE, "Close"=FALSE}, "DB - [AMS].[Execute].[Message] Enum"=DB_-_[AMS].[Execute].[Message]_Enum."UPDATE", "AMS Execute Message ColNames"=w301, "<Data> (0xFFFE autodetect)"=w297, "error in (no error)"=w295, "<SIGN>"="=", "[MessageNo]"=w277) -> ("connection reference"=w294:T5, "SUMMARY"=w293:errorcluster)  [unwired: 4 in, 2 out]
            }
          }
          frame "1" {
            w380 = 13  # [SmsDeliveredStatusCode]
            w381 = 12  # [SmsProcessStatusCode]
            w385 = 12  # String1 to String12
            # "SMS                                                                                     SMS                                                                                     SMS                                                                                     SMS                                                                                     SMS                                                                                     SMS                                                                                     SMS"
            n134 = Index Array(array=w387, index (row)=0) -> (element=w382:string[])  [unwired: 1 in]
            n135 = local read "Simulate Parameters"() -> (w359:T1)
            n136 = Index Array(array=w382, index #1=w381, index #2=w380) -> (element #1=w358:string)  [unwired: 1 out]
            n137 = Unbundle By Name(w359) -> ("Simulate Send SMS"=w361:bool, "Simulate Stringx [Unicode]"=w360:bool)
            n138 = for {
              N: w385 -> [_]
              tunnel: w382 -> [w485] mode=indexing
              tunnel: w368 -> [w486]
              shift-right: [w483] -> w384
              shift-left: "" -> [w482]
              tunnel: w360 -> [w481]
              w489 = FALSE  # Shouldn't have unicode here
              n139 = call "String - Search for [[  ]].vi"("String"=w485, "Strip \\00 (Unicode)"=w489) -> ("matched string"=w487:string, "Found"=w488:bool)  [unwired: 6 in, 2 out]
              n140 = case shown="True" w488 {
                tunnel: w487 -> [_ w496]
                tunnel: w486 -> [_ w494]
                tunnel: w485 -> [w490 w493]
                tunnel: [w490 w492] -> w484
                tunnel: w481 -> [_ w491]
                frame False {
                }
                frame True {
                  # "[[ColName]] Found\nGet Column Index\nGet Value"
                  n141 = To Upper Case(1:w496) -> (0:w495:string)
                  n142 = case shown="\"False\", Default" w495 {
                    tunnel: w494 -> [_ w498 _ _]
                    tunnel: [w497 w498 w501 w508] -> w492
                    tunnel: w493 -> [w497 _ _ _]
                    tunnel: w491 -> [_ _ _ w504]
                    frame "False", Default {
                    }
                    frame "MESSAGE.MOBILENOS" {
                    }
                    frame "MESSAGETEMPLATE.SUBJECT" {
                      n143 = local read "[MessageTemplate.Subject] Unicode"() -> (w503:string)
                      n144 = call "String - Remove Front 0xFFFEs.vi"("Sting IN"=w503) -> ("String OUT"=w502:string)  [unwired: 10 in]
                      n145 = Search and Replace String(replace all?=TRUE ("replace all? (F)"), input string=w502, search string="\u0000" ("input string")) -> (result string=w501:string)  [unwired: 5 in, 3 out]
                    }
                    frame "MESSAGETEMPLATE.STRINGS" {
                      n146 = local read "Stringx [Unicode]"() -> (w506:string)
                      n147 = Select(t="Simulate Stringx [Unicode]", s=w504, f=w506) -> (s? t:f=w505:string)
                      n148 = local write "Stringx [Unicode]"(w505) -> ()
                      n149 = call "String - String to Bytes (Swapped).vi"("String"=w505) -> ("Sting Out"=w508:string)  [unwired: 10 in]
                    }
                  }
                }
              }
              n150 = Concatenate Strings(w482, w484) -> (w483:string)
            }
            "SMSString" <- w384
            n151 = while {
              tunnel: w361 -> [w460]
              tunnel: w384 -> [w415]
              tunnel: w358 -> [w459]
              tunnel: w379 -> [w458]
              tunnel: w378 -> [w456]
              tunnel: w377 -> [w454]
              tunnel: w376 -> [w453]
              tunnel: w375 -> [w452]
              tunnel: w374 -> [w407]
              tunnel: w373 -> [w449]
              tunnel: w372 -> [w414]
              tunnel: [w417] -> w371
              tunnel: [w394] -> w370
              tunnel: w369 -> [w424]
              tunnel: w368 -> [w413]
              tunnel: w367 -> [w433]
              tunnel: w366 -> [w426]
              tunnel: [w402] -> w365
              tunnel: w364 -> [w401]
              tunnel: [w397] -> w363
              tunnel: [w389] -> w362
              i -> [w442]
              stop <- w403 stop-if-true
              w416 = T4[] [enum."[SmsContent]", enum."[LastAttemptedCommMed]", enum."[LastAttemptedNo]", enum."[LastAttemptedOn]", enum."[IsSmsSent]"] items=["[MessageNo]", "[LanguageId]", "[SoftwareSolutionId]", "[SoftwareSolutionName]", "[PlantId]", "[SystemId]", "[StationId]", "[MessageLogNo]", "[ReceivedOn]", "[MessageCode]", "[ShortDescription]", "[Message]", "[SmsMessage]", "[SuppMessage1]", "[SuppMessage2]", "[SuppMessage3]", "[TransactionNo]", "[TransactionRunNo]", "[MessageInitiator]", "[Remarks]", "[MsgCreatedOn]", "[IsToSendSms]", "[IsToSendEmail]", "[IsToSendCommMedium1]", "[IsToSendCommMedium2]", "[SmsContent]", "[EmailContent]", "[CommMed1Content]", "[CommMed2Content]", "[MobileNos]", "[EmailAddresses]", "[CommMedium1Ids]", "[CommMedium2Ids]", "[LastAttemptedCommMed]", "[LastAttemptedNo]", "[LastAttemptedOn]", "[IsSmsSent]", "[IsEmailSent]", "[IsCommMedium1Sent]", "[IsCommMedium2Sent]", "[OverallSentStatus]", "[StatusUpdatedOn]", "[IsArchived]"] ("AMS Execute Message ColNames")
              w430 = 0 ("index (row)")
              n152 = case shown="False" w460 {
                tunnel: w415 -> [w474 _]
                tunnel: w459 -> [w470 _]
                tunnel: [w468 w480] -> w402
                tunnel: [w464 w475] -> w423
                tunnel: [w467 w478] -> w443
                frame False {
                  w465 = 0  # MobileNo
                  w471 = 2  # StatusId
                  w472 = 1  # MessageRefNo
                  # "Don't Simulate\nUse REAL!!"
                  n153 = call "Comm - Send SMS.vi"("url"=w474) -> ("error out"=→"SMS":errorcluster, "MobileNo, MessageRefNo, StatusId"=w473:string[])  [unwired: 9 in]
                  n154 = Index Array(array=w473, index #1=w465, index #2=w472, index #3=w471) -> (element #2=w464:string, element #3=w467:string)  [unwired: 1 out]
                  n155 = Equal?(x=w467, y=w470) -> (x = y?=w468:bool)
                  "Message Delivered OK" <- w468
                  n156 = Wait Until Next ms Multiple(millisecond multiple=u32 1) -> ()  [unwired: 1 out]
                }
                frame True {
                  w480 = TRUE
                  # "Simulate"
                  n157 = Tick Count (ms)() -> (millisecond timer value=w476:u32)
                  n158 = Number To Decimal String(number=w476) -> (decimal integer string=w475:string)  [unwired: 1 in]
                  n159 = Select(t="200" ("element"), s=w480, f="501" ("element")) -> (s? t:f=w478:string)
                }
              }
              n160 = global read "Global AMS.vi" "Date Time Format"() -> (w441:string)
              n161 = Format Date/Time String(time format string (%c)=w441) -> (date/time string=w388:string)  [unwired: 2 in]
              n162 = Equal?(x=w442, y=w458) -> (x = y?=w457:bool)
              n163 = Search 1D Array(1D array=w407, element=DB_-_[AMS].[Execute].[Message]_ColNames."[MessageNo]" ("[AMS].[Execute].[Message] ColNames")) -> (index of element=w450:i32)  [unwired: 1 in]
              n164 = Search 1D Array(1D array=w407, element=DB_-_[AMS].[Execute].[Message]_ColNames."[PlantId]" ("[AMS].[Execute].[Message] ColNames")) -> (index of element=w444:i32)  [unwired: 1 in]
              n165 = Search 1D Array(1D array=w407, element=DB_-_[AMS].[Execute].[Message]_ColNames."[MessageNo]" ("[AMS].[Execute].[Message] ColNames")) -> (index of element=w405:i32)  [unwired: 1 in]
              n166 = Number To Decimal String(number=w442) -> (decimal integer string=w391:string)  [unwired: 1 in]
              n167 = Index Array(array=w449, index #1=w450, index #2=w444, index #3=w405) -> (element #1=w447:string, element #2=w425:string, element #3=w389:string)
              n168 = Select(t="1", s=w402, f="0") -> (s? t:f=w412:string)
              n169 = Build Array(w447, w414, w425, w424, w413, w423, w443, w391, w388, w412, "", "SYSDATETIME()", "0" ("element")) -> (w445:string[])
              n170 = call "DB - Array to Values.vi"("Array (0xFFFE autodetect)"=w445) -> ("<Values>"=w446:string)  [unwired: 10 in]
              n171 = Search and Replace String(input string=w454, search string="<Values>", replace string=w446) -> (result string=w400:string)  [unwired: 5 in, 3 out]
              n172 = Or(x=w402, y=w457) -> (x .or. y?=w403:bool)
              n173 = call "DB - T-SQL Query.vi"("error in (no error)"=w452, "T-SQL"=w400, "connection reference"=w453) -> ("error out"=w434:errorcluster, "connection reference"=w435:T5)  [unwired: 6 in, 1 out]
              "AMS.Execute.MessageProcessLog" <- w434
              n174 = case shown="False" w403 {
                tunnel: w456 -> [w462 _]
                frame False {
                  # "Wait if FALSE"
                  n175 = Multiply(x=1000, y=w462) -> (x*y=w463:i32)
                  n176 = Wait (ms)(milliseconds to wait=w463) -> ()  [unwired: 1 out]
                }
                frame True {
                }
              }
              n177 = Search and Replace String(input string=w433, search string="<MRN>", replace string=w423) -> (result string=w399:string)  [unwired: 5 in, 3 out]
              n178 = call "DB - T-SQL Query.vi"("error in (no error)"=w434, "T-SQL"=w399, "connection reference"=w435) -> ("error out"=w393:errorcluster, "2D data"=w431:string[][], "connection reference"=w429:T5)  [unwired: 6 in]
              "AMS.Execute.MessageProcessLog 2" <- w393
              n179 = Index Array(array=w431, index (row)=w430, index (col)=w430) -> (element=w422:string)
              n180 = Build Array(w425, w424, w423, w422, "0" ("element")) -> (w420:string[])
              n181 = call "DB - Array to Values.vi"("Array (0xFFFE autodetect)"=w420) -> ("<Values>"=w428:string)  [unwired: 10 in]
              n182 = Search and Replace String(input string=w426, search string="<Values>", replace string=w428) -> (result string=w398:string)  [unwired: 5 in, 3 out]
              n183 = call "DB - T-SQL Query.vi"("error in (no error)"=w393, "T-SQL"=w398, "connection reference"=w429) -> ("error out"=w395:errorcluster, "connection reference"=w418:T5)  [unwired: 6 in, 1 out]
              "AMS.Execute.SmsRefNoLogRelation" <- w395
              n184 = local read "Stringx [Unicode]"() -> (w390:string)
              n185 = local write "[MessageNo]"(w389) -> ()
              n186 = call "String - Add BOM if IsUnicode.vi"("target length (65535)"=500, "Input is Unicode (varbinary)?"=TRUE ("IsUnicode?"), "String IN"=w390) -> ("BOM Added"=w411:string)  [unwired: 8 in]
              n187 = Build Array(w411, w414, w391, w388, w412) -> (w408:string[])
              n188 = call "DB - [AMS].[Execute].[Message].vi"("connection reference"=w418, "DB Connection"=T6 {"Open"=FALSE, "Close"=FALSE}, "DB - [AMS].[Execute].[Message] Enum"=DB_-_[AMS].[Execute].[Message]_Enum."UPDATE", "AMS Execute Message ColNames"=w416, "<Data> (0xFFFE autodetect)"=w408, "error in (no error)"=w395, "<SIGN>"="=", "[MessageNo]"=w389) -> ("connection reference"=w417:T5, "SQL Statement"=w392:string, "SUMMARY"=w394:errorcluster)  [unwired: 4 in, 1 out]
              "AMS.Execute.Message" <- w394
              n189 = Build Array(w401, w400, w399, w398, w392) -> (w397:string[])
            }
          }
        }
      }
      frame Error {
        n190 = Build Array(w510) -> (w509:string[])
      }
    }
  }
  n191 = disable-structure shown="Enabled" {
    disable-tunnel: w13 -> [w521 w525]
    disable-tunnel: [w520 w525] -> w12
    disable-tunnel: w11 -> [w519 w524]
    disable-tunnel: [w518 w524] -> w10
    disable-tunnel: w8 -> [w516 _]
    disable-tunnel: w5 -> [w514 _]
    frame Disabled {
      w517 = T4[] [enum."[OverallSentStatus]", enum."[StatusUpdatedOn]"] items=["[MessageNo]", "[LanguageId]", "[SoftwareSolutionId]", "[SoftwareSolutionName]", "[PlantId]", "[SystemId]", "[StationId]", "[MessageLogNo]", "[ReceivedOn]", "[MessageCode]", "[ShortDescription]", "[Message]", "[SmsMessage]", "[SuppMessage1]", "[SuppMessage2]", "[SuppMessage3]", "[TransactionNo]", "[TransactionRunNo]", "[MessageInitiator]", "[Remarks]", "[MsgCreatedOn]", "[IsToSendSms]", "[IsToSendEmail]", "[IsToSendCommMedium1]", "[IsToSendCommMedium2]", "[SmsContent]", "[EmailContent]", "[CommMed1Content]", "[CommMed2Content]", "[MobileNos]", "[EmailAddresses]", "[CommMedium1Ids]", "[CommMedium2Ids]", "[LastAttemptedCommMed]", "[LastAttemptedNo]", "[LastAttemptedOn]", "[IsSmsSent]", "[IsEmailSent]", "[IsCommMedium1Sent]", "[IsCommMedium2Sent]", "[OverallSentStatus]", "[StatusUpdatedOn]", "[IsArchived]"] ("AMS Execute Message ColNames")
      n192 = call "DB - [AMS].[Execute].[Message].vi"("connection reference"=w521, "DB Connection"=T6 {"Open"=FALSE, "Close"=FALSE}, "DB - [AMS].[Execute].[Message] Enum"=DB_-_[AMS].[Execute].[Message]_Enum."UPDATE", "AMS Execute Message ColNames"=w517, "<Data> (0xFFFE autodetect)"=w516, "error in (no error)"=w519, "<SIGN>"="=", "[MessageNo]"=w514) -> ("connection reference"=w520:T5, "SUMMARY"=w518:errorcluster)  [unwired: 4 in, 2 out]
    }
    frame Enabled {
    }
  }
  "SUMMARY" <- w10
  "connection reference" <- w12
  n193 = flat-sequence {
    tunnel: w9 -> [w533]
    tunnel: [w526] -> w8
    frame #0 {
      n194 = global read "Global AMS.vi" "Date Time Format"() -> (w532:string)
      n195 = And Array Elements(Boolean array=w533) -> (logical AND=w531:bool)
      "All SMS/Email Delivered OK" <- w531
      n196 = Select(t="1", s=w531, f="0") -> (s? t:f=w528:string)
      n197 = Format Date/Time String(time format string (%c)=w532) -> (date/time string=w527:string)  [unwired: 2 in]
      n198 = Build Array(w528, w527) -> (w526:string[])
      "Final Message Delivered OK" <- w533
    }
  }
  n199 = Build Array (concatenate)(w55, w54, w7) -> (→"SQL":string[])
  n200 = case shown="True" w88 {
    tunnel: w12 -> [_ w535]
    tunnel: w10 -> [_ _]
    frame False {
      # "Ref Connected"
    }
    frame True {
      # "CLOSE"
      n201 = call <vilib>:"DB Tools Close Connection.vi"("connection reference"=w535) -> ("error out"=→"Close":errorcluster)  [unwired: 6 in]
    }
  }
  n202 = global write "Global SRTRS.vi" "DB Error"(w10) -> ()
